vi "Global stato profilo.vi"() -> ()   [LabVIEW 2019]
panel:
  out "STATO PROFILO":T1
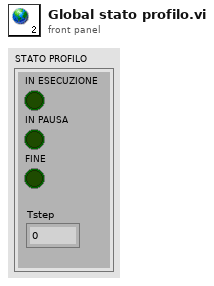
[diagram p1: front panel]
types:
  T1 = cluster{"IN ESECUZIONE":bool, "IN PAUSA":bool, "FINE":bool, "Tstep":dbl}
diagram:
